vi "Get Spec.vi"(4 "NumRows":u32, 6 "Spec in":string[][](array[string]), 7 "Spec Ref.":refnum<vi>, 8 "error in":errorcluster caption="에러 입력(에러 없음)", 9 "Condition in":string[][](array[string]), 10 "Resolution in":string[][](array[string]), 11 "Func_ext":string) -> (0 "error out":errorcluster caption="에러 출력", 1 "Data Out":string[][](array[string]), 2 "Spec Out":string[][](array[string]), 3 "Func_ext Out":string, 5 "Spec (Default)":string[][](array[string]))   [LabVIEW 2020]
uses:
  Controls/Cmd_Var Data IO.ctl
  Variables/Global_Cal Info.vi
  Public/Polymorph/Data Class_2D Str.vi
panel:
  out "match spec":string[][](array[string])
  # "FUNC, FUNC_EXT, FUNC_CON, C1_VAL, C1_UNIT, RANGE_VAL, RANGE_UNIT"
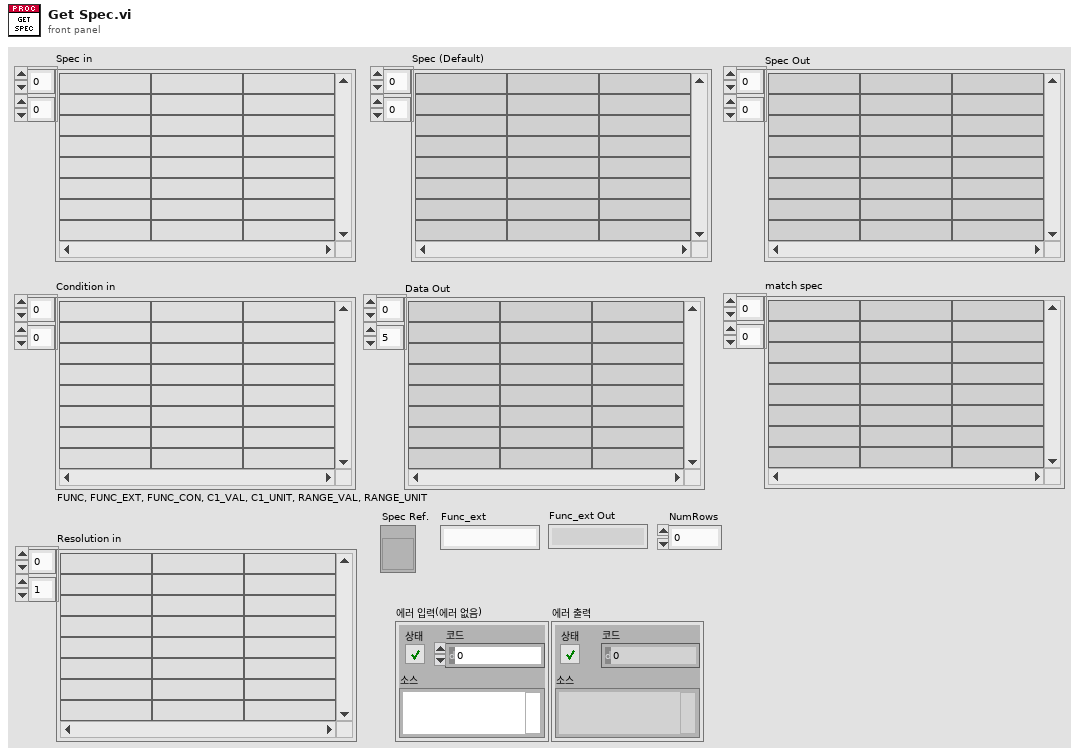
[diagram p1: front panel]
types:
  T1 = typedef "Cmd_Var Data IO.ctl" = enum16{"Condition", "Condition Default", "Condition_Temp", "Resolution", "Resolution Default", "Resolution Old", "Spec", "Spec Default", "Spec Old", "Spec Temp", "Result", "Result2", "Result3", "Result_Temp", "Result_ADJ", "Result_ADJ2", "STD1", "STD2", "STD3", "STD4", "STD5", "STD Temp", "CMC", "CMC Default"}
  T2 = cluster{"세부분류코드":string, "형식":string, "옵션":string, "측정기명":string, "EXCEL파일명":string, "TEMP":string}
  T3 = typedef "Clst_Cal Info Global.ctl" = cluster{"등록번호":string, "의뢰기관":string, "기기명":string, "제작회사":string, "형식":string, "기기번호":string, "소분류코드":string, "세부분류코드":string, "교정주기":string, "접수번호":string, "교정일자":string, "교정절차서 1":string, "교정절차서 2":string, "교정절차서 3":string, "접수확인자":string, "인증교정자":string, "기술책임자":string, "KOLAS 유무":string, "진행상태":string, "의뢰기관코드":string, "입고형태":string, "영문성적서?":bool, "합불판정?":bool, "부록?":bool, "절차서번호 1":string, "절차서번호 2":string, "절차서번호 3":string, "교정방식":string, "부서명":string}
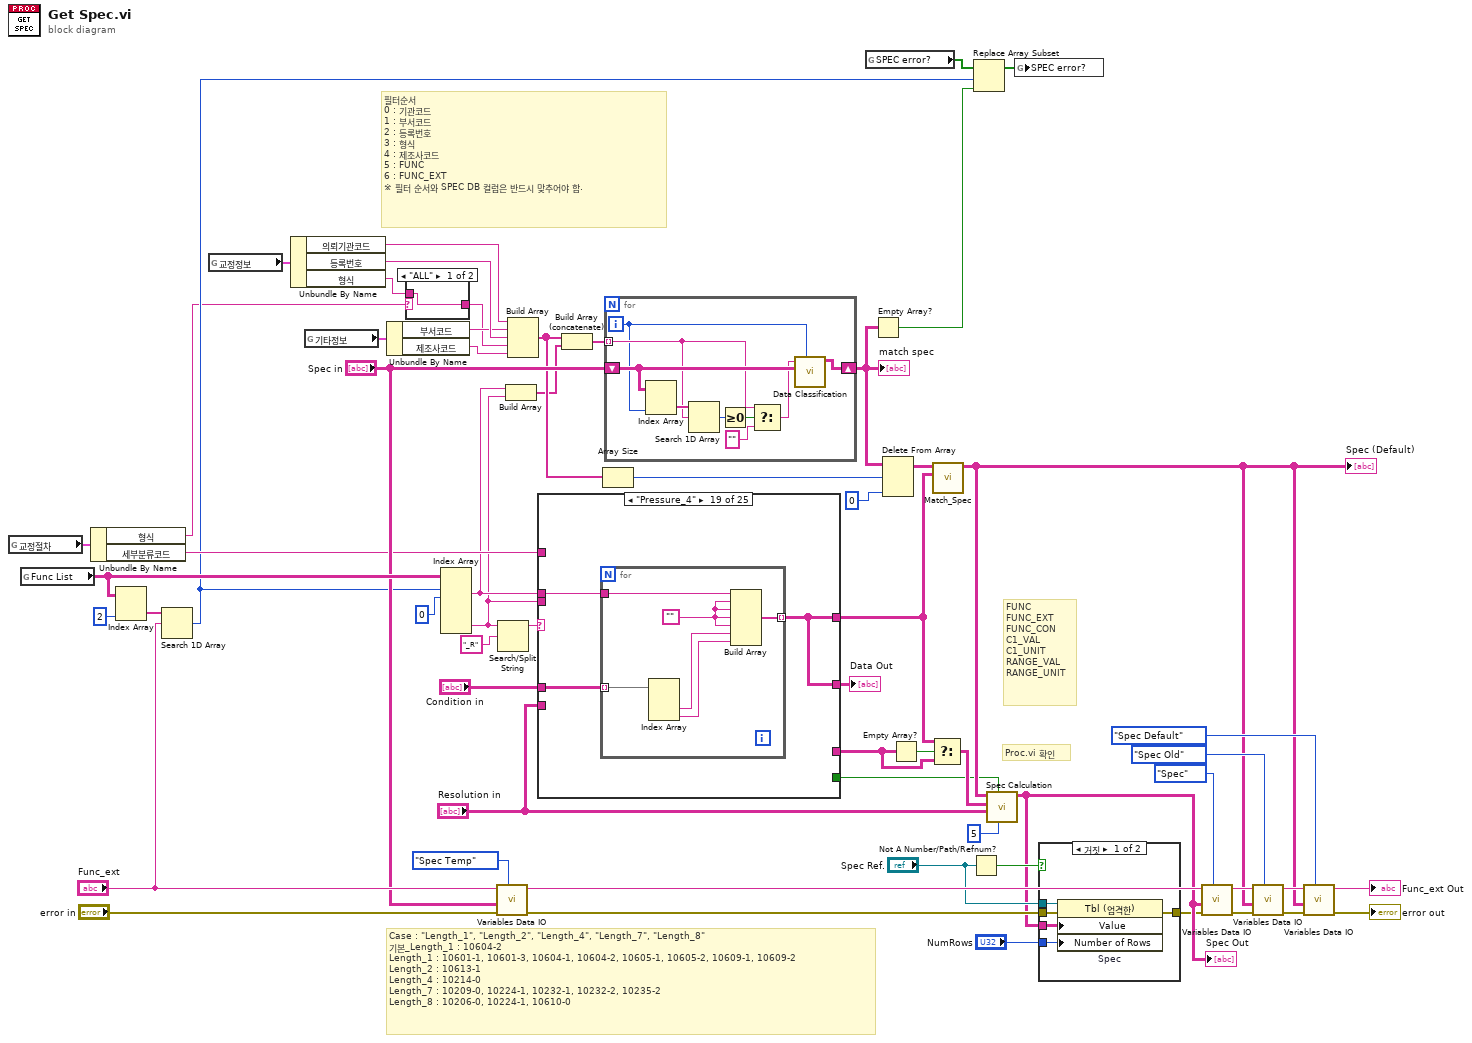
[diagram p0: block diagram]
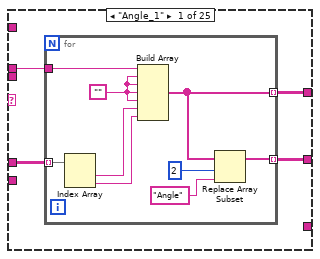
[diagram p4: hidden frame]
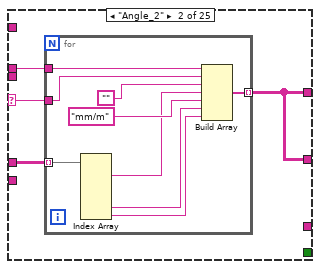
[diagram p5: hidden frame]
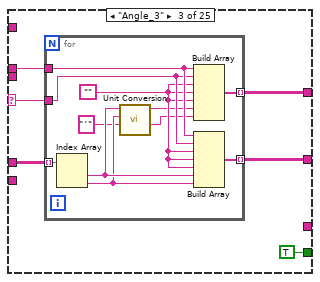
[diagram p6: hidden frame]
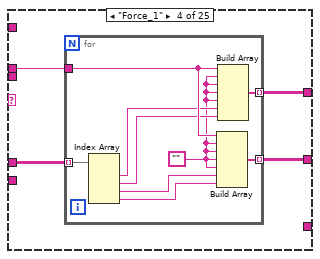
[diagram p7: hidden frame]
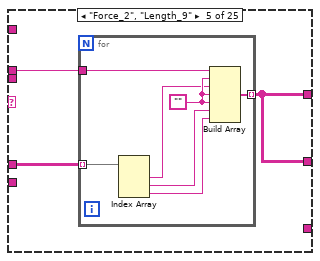
[diagram p8: hidden frame]
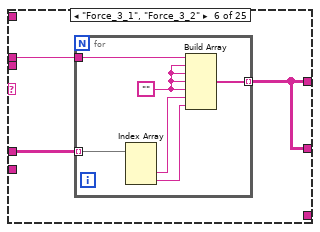
[diagram p9: hidden frame]
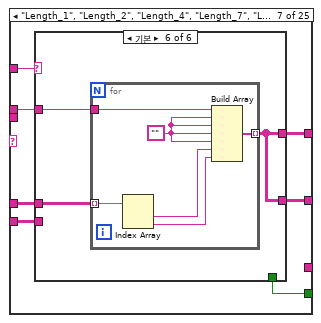
[diagram p10: hidden frame]
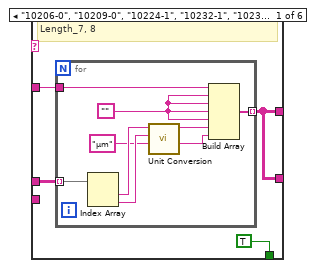
[diagram p11: hidden frame]
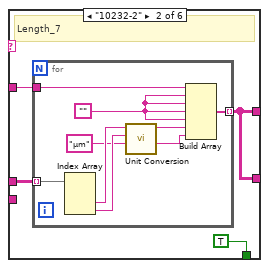
[diagram p12: hidden frame]
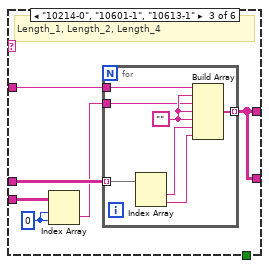
[diagram p13: hidden frame]
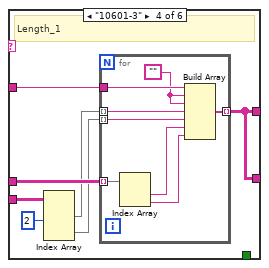
[diagram p14: hidden frame]
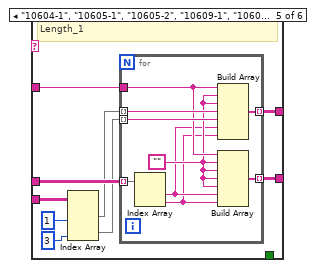
[diagram p15: hidden frame]
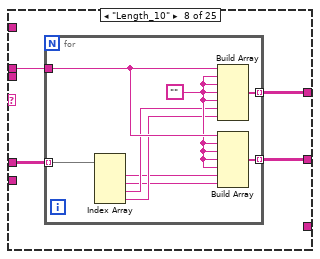
[diagram p16: hidden frame]
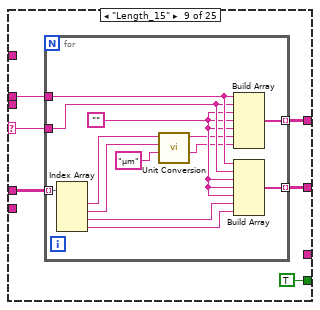
[diagram p17: hidden frame]
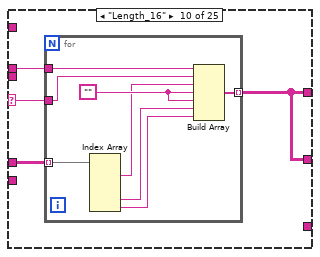
[diagram p18: hidden frame]
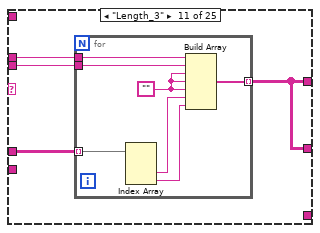
[diagram p19: hidden frame]
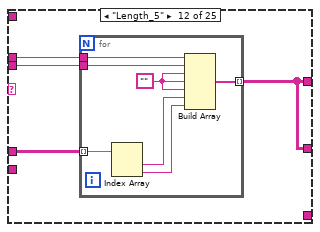
[diagram p20: hidden frame]
diagram:
  # "Proc.vi 확인"
  # "Case : \"Length_1\", \"Length_2\", \"Length_4\", \"Length_7\", \"Length_8\" \n기본_Length_1 : 10604-2\nLength_1 : 10601-1, 10601-3, 10604-1, 10604-2, 10605-1, 10605-2, 10609-1, 10609-2\nLength_2 : 10613-1\nLength_4 : 10214-0\nLength_7 : 10209-0, 10224-1, 10232-1, 10232-2, 10235-2\nLength_8 : 10206-0, 10224-1, 10610-0"
  # "필터순서\n0 : 기관코드\n1 : 부서코드\n2 : 등록번호\n3 : 형식\n4 : 제조사코드\n5 : FUNC\n6 : FUNC_EXT\n※ 필터 순서와 SPEC DB 컬럼은 반드시 맞추어야 함."
  # "FUNC\nFUNC_EXT\nFUNC_CON\nC1_VAL\nC1_UNIT\nRANGE_VAL\nRANGE_UNIT"
  n1 = global read "Global_Cal Info.vi" "교정절차"() -> (w59:T2)
  n2 = global read "Global_Cal Info.vi" "Func List"() -> (w48:string[][])
  n3 = Unbundle By Name(w59) -> ("형식"=w2:string, "세부분류코드"=w30:string)
  n4 = Index Array(array=w48, index (col)=2 ("비활성화된 인덱스 (열)")) -> (element=w50:string[])  [unwired: 1 in]
  n5 = Search 1D Array(1D array=w50, element="Func_ext") -> (index of element=w6:i32)  [unwired: 1 in]
  n6 = global read "Global_Cal Info.vi" "교정정보"() -> (w60:T3)
  n7 = Unbundle By Name(w60) -> ("의뢰기관코드"=w20:string, "등록번호"=w26:string, "형식"=w1:string)
  n8 = global read "Global_Cal Info.vi" "기타정보"() -> (w25:cluster{"부서코드":string, "제조사코드":string})
  n9 = Unbundle By Name(w25) -> ("부서코드"=w24:string, "제조사코드"=w23:string)
  n10 = case shown="\"ALL\"" w2 {
    selector: w2 -> [_ w62]
    tunnel: [w61 w62] -> w3
    tunnel: w1 -> [w61 _]
    frame "ALL" {
    }
    frame Default {
    }
  }
  n11 = Index Array(array=w48, index (row) #1=w6, index (col) #1=0 ("비활성화된 인덱스 (열)")) -> (element #1=w19:string, element #3=w18:string)  [unwired: 4 in, 1 out]
  n12 = call "Variables Data IO.vi"("Select"=Cmd_Var_Data_IO."Spec Temp", "error in"="error in", "Data In"="Spec in", "Func_ext"="Func_ext") -> ("error out"=w38:errorcluster, "Func_ext Out"=w36:string)  [unwired: 5 in, 1 out]
  n13 = Search/Split String(string=w18, search string/char (-)="_R" ("검색 문자열/문자 (-)")) -> (substring before match=w32:string)  [unwired: 1 in, 2 out]
  n14 = Build Array(w19, w18) -> (w16:string[])
  n15 = Build Array(w20, w24, w26, w3, w23) -> (w21:string[])
  n16 = case shown="\"Pressure_4\"" w32 {
    selector: w32 -> [_ w77 w92 _ _ _ _ _ w242 w259 _ _ w294 _ w322 _ _ _ _ w415 w431 w446 w462 w478 _]
    tunnel: "Condition in" -> [w66 w79 w94 w109 w121 w131 w144 w229 w244 w261 w273 w284 w296 w310 w324 w332 w342 w354 w405 w417 w433 w448 w464 w480 w494]
    tunnel: w19 -> [w65 w78 w93 w108 w120 w130 w143 w228 w243 w260 w272 w283 w295 w309 w323 w331 w341 w353 w404 w416 w432 w447 w463 w479 w493]
    tunnel: [w64 w76 w89 w107 w119 w129 w142 w227 w240 w258 w271 w282 w293 w307 w321 w330 w340 w351 w403 w413 w430 w443 w461 w476 w492] -> w13
    tunnel: [w63 w76 w91 w106 w119 w129 w139 w226 w241 w258 w271 w282 w293 w308 w321 w330 w340 w350 w403 w414 w430 w445 w461 w475 w492] -> w31
    tunnel: w30 -> [_ _ _ _ _ _ w140 _ _ _ _ _ _ _ _ _ _ w352 _ _ _ _ _ _ _]
    tunnel: "Resolution in" -> [_ _ _ _ _ _ w141 _ _ _ _ _ _ _ _ _ _ _ _ _ _ _ _ w477 _]
    tunnel: w18 -> [_ _ _ _ _ _ _ _ _ _ w270 w281 _ _ _ _ _ _ _ _ _ _ _ _ _]
    tunnel: [_ _ TRUE _ _ _ w138 _ TRUE _ _ _ TRUE _ _ _ _ _ _ _ TRUE TRUE _ _ _] -> w4
    tunnel: [_ _ _ _ _ _ _ _ _ _ _ _ _ _ _ _ _ _ _ w412 _ _ w460 _ _] -> w11
    frame "Angle_1" {
      n17 = for {
        tunnel: w66 -> [w75] mode=indexing
        tunnel: [w70] -> w64 mode=indexing
        tunnel: w65 -> [w74]
        tunnel: [w69] -> w63 mode=indexing
        w71 = ""
        n18 = Index Array(array=w75) -> (element #1=w72:string, element #2=w73:string)  [unwired: 2 in]
        n19 = Build Array(w74, w71, w71, w71, w71, w72, w73) -> (w70:string[])
        n20 = Replace Array Subset(array=w70, new element="Angle" ("새 원소/부분배열"), index=2 ("인덱스")) -> (w69:string[])
      }
    }
    frame "Angle_2" {
      n21 = for {
        tunnel: w79 -> [w88] mode=indexing
        tunnel: [w87] -> w76 mode=indexing
        tunnel: w78 -> [w86]
        tunnel: w77 -> [w85]
        n22 = Index Array(array=w88) -> (element #1=w82:string, element #5=w80:string, element #6=w81:string)  [unwired: 6 in, 3 out]
        n23 = Build Array(w86, w85, "", w82, "mm/m" ("원소"), w80, w81) -> (w87:string[])
      }
    }
    frame "Angle_3" {
      n24 = for {
        tunnel: w94 -> [w105] mode=indexing
        tunnel: [w104] -> w89 mode=indexing
        tunnel: w93 -> [w103]
        tunnel: [w102] -> w91 mode=indexing
        tunnel: w92 -> [w101]
        w100 = ""
        n25 = Index Array(array=w105) -> (element #1=w97:string, element #2=w96:string)  [unwired: 2 in]
        n26 = call "Unit Conversion.vi"("환산단위"="´", "입력단위"=w96, "입력값"=w97) -> ("환산단위"=w98:string, "환산값 (string)"=w99:string)  [unwired: 3 in, 4 out]
        n27 = Build Array(w103, w101, w100, w100, w100, w99, w98) -> (w104:string[])
        n28 = Build Array(w103, w101, w100, w100, w100, w97, w96) -> (w102:string[])
      }
    }
    frame "Force_1" {
      n29 = for {
        tunnel: w109 -> [w118] mode=indexing
        tunnel: [w117] -> w107 mode=indexing
        tunnel: w108 -> [w115]
        tunnel: [w116] -> w106 mode=indexing
        w110 = ""
        n30 = Index Array(array=w118) -> (element #1=w112:string, element #2=w111:string, element #3=w114:string, element #4=w113:string)  [unwired: 4 in]
        n31 = Build Array(w115, w110, w110, w110, w110, w114, w113) -> (w116:string[])
        n32 = Build Array(w115, w110, w110, w110, w110, w112, w111) -> (w117:string[])
      }
    }
    frame "Force_2", "Length_9" {
      n33 = for {
        tunnel: w121 -> [w128] mode=indexing
        tunnel: [w127] -> w119 mode=indexing
        tunnel: w120 -> [w126]
        w125 = ""
        n34 = Index Array(array=w128) -> (element #1=w124:string, element #2=w123:string, element #3=w122:string)  [unwired: 3 in]
        n35 = Build Array(w126, w125, w124, w125, w125, w123, w122) -> (w127:string[])
      }
    }
    frame "Force_3_1", "Force_3_2" {
      n36 = for {
        tunnel: w131 -> [w137] mode=indexing
        tunnel: [w136] -> w129 mode=indexing
        tunnel: w130 -> [w135]
        w132 = ""
        n37 = Index Array(array=w137) -> (element #2=w133:string, element #3=w134:string)  [unwired: 3 in, 1 out]
        n38 = Build Array(w135, w132, w132, w132, w132, w133, w134) -> (w136:string[])
      }
    }
    frame "Length_1", "Length_2", "Length_4", "Length_7", "Length_8" {
      n39 = case shown="기본" w140 {
        tunnel: w144 -> [w148 w161 w176 w190 w207 w219]
        tunnel: w143 -> [w147 w160 w175 w189 w206 w218]
        tunnel: [w146 w159 w171 w184 w205 w217] -> w142
        tunnel: w141 -> [_ _ w174 w188 w204 _]
        tunnel: [w146 w159 w171 w184 w199 w217] -> w139
        tunnel: [TRUE TRUE _ _ _ _] -> w138
        frame "10206-0", "10209-0", "10224-1", "10232-1", "10235-2", "10610-0" {
          # "Length_7, 8"
          n40 = for {
            tunnel: w148 -> [w157] mode=indexing
            tunnel: [w156] -> w146 mode=indexing
            tunnel: w147 -> [w155]
            w154 = ""
            n41 = Index Array(array=w157) -> (element #1=w153:string, element #2=w152:string)  [unwired: 2 in]
            n42 = call "Unit Conversion.vi"("환산단위"="μm", "입력단위"=w152, "입력값"=w153) -> ("환산단위"=w149:string, "환산값 (string)"=w150:string)  [unwired: 3 in, 4 out]
            n43 = Build Array(w155, w154, w154, w154, w154, w150, w149) -> (w156:string[])
          }
        }
        frame "10232-2" {
          # "Length_7"
          n44 = for {
            tunnel: w161 -> [w170] mode=indexing
            tunnel: [w169] -> w159 mode=indexing
            tunnel: w160 -> [w168]
            w167 = ""
            n45 = Index Array(array=w170) -> (element #2=w166:string, element #3=w165:string)  [unwired: 3 in, 1 out]
            n46 = call "Unit Conversion.vi"("환산단위"="μm", "입력단위"=w165, "입력값"=w166) -> ("환산단위"=w162:string, "환산값 (string)"=w163:string)  [unwired: 3 in, 4 out]
            n47 = Build Array(w168, w167, w167, w167, w167, w163, w162) -> (w169:string[])
          }
        }
        frame "10214-0", "10601-1", "10613-1" {
          w173 = 0 ("인덱스 (행)")
          # "Length_1, Length_2, Length_4"
          n48 = Index Array(array=w174, index (row)=w173, index (col)=w173) -> (element=w172:string)
          n49 = for {
            tunnel: w176 -> [w183] mode=indexing
            tunnel: [w182] -> w171 mode=indexing
            tunnel: w175 -> [w181]
            tunnel: w172 -> [w177]
            w178 = ""
            n50 = Index Array(array=w183) -> (element #1=w179:string, element #2=w180:string)  [unwired: 2 in]
            n51 = Build Array(w181, w178, w177, w178, w178, w179, w180) -> (w182:string[])
          }
        }
        frame "10601-3" {
          # "Length_1"
          n52 = Index Array(array=w188, index (col) #1=2 ("비활성화된 인덱스 (열)")) -> (element #1=w186:string[], element #2=w185:string[])  [unwired: 3 in]
          n53 = for {
            tunnel: w190 -> [w198] mode=indexing
            tunnel: [w197] -> w184 mode=indexing
            tunnel: w189 -> [w196]
            tunnel: w186 -> [w192] mode=indexing
            tunnel: w185 -> [w191] mode=indexing
            w193 = ""
            n54 = Index Array(array=w198) -> (element #1=w194:string, element #2=w195:string)  [unwired: 2 in]
            n55 = Build Array(w196, w193, w193, w192, w191, w194, w195) -> (w197:string[])
          }
        }
        frame "10604-1", "10605-1", "10605-2", "10609-1", "10609-2" {
          # "Length_1"
          n56 = Index Array(array=w204, index (col) #1=1 ("비활성화된 인덱스 (열)"), index (col) #2=3 ("인덱스 (열)")) -> (element #1=w202:string[], element #2=w201:string[])  [unwired: 2 in]
          n57 = for {
            tunnel: w207 -> [w216] mode=indexing
            tunnel: [w215] -> w205 mode=indexing
            tunnel: w206 -> [w212]
            tunnel: w202 -> [w214] mode=indexing
            tunnel: w201 -> [w213] mode=indexing
            tunnel: [w208] -> w199 mode=indexing
            w211 = ""
            n58 = Index Array(array=w216) -> (element #1=w210:string, element #2=w209:string)  [unwired: 2 in]
            n59 = Build Array(w212, w211, w211, w214, w213, w210, w209) -> (w215:string[])
            n60 = Build Array(w212, w211, w211, w211, w211, w210, w209) -> (w208:string[])
          }
        }
        frame Default {
          n61 = for {
            tunnel: w219 -> [w225] mode=indexing
            tunnel: [w224] -> w217 mode=indexing
            tunnel: w218 -> [w223]
            w221 = ""
            n62 = Index Array(array=w225) -> (element #1=w220:string, element #2=w222:string)  [unwired: 2 in]
            n63 = Build Array(w223, w221, w221, w221, w221, w220, w222) -> (w224:string[])
          }
        }
      }
    }
    frame "Length_10" {
      n64 = for {
        tunnel: w229 -> [w238] mode=indexing
        tunnel: [w237] -> w227 mode=indexing
        tunnel: w228 -> [w236]
        tunnel: [w235] -> w226 mode=indexing
        w234 = ""
        n65 = Index Array(array=w238) -> (element #1=w231:string, element #2=w230:string, element #3=w233:string, element #4=w232:string)  [unwired: 4 in]
        n66 = Build Array(w236, w234, w234, w234, w234, w233, w232) -> (w237:string[])
        n67 = Build Array(w236, w234, w234, w234, w234, w231, w230) -> (w235:string[])
      }
    }
    frame "Length_15" {
      n68 = for {
        tunnel: w244 -> [w257] mode=indexing
        tunnel: [w256] -> w240 mode=indexing
        tunnel: w243 -> [w255]
        tunnel: [w254] -> w241 mode=indexing
        tunnel: w242 -> [w253]
        w252 = ""
        n69 = Index Array(array=w257) -> (element #1=w249:string, element #2=w248:string, element #3=w251:string, element #4=w250:string)  [unwired: 4 in]
        n70 = call "Unit Conversion.vi"("환산단위"="μm", "입력단위"=w248, "입력값"=w249) -> ("환산단위"=w245:string, "환산값 (string)"=w246:string)  [unwired: 3 in, 4 out]
        n71 = Build Array(w255, w253, w252, w252, w252, w246, w245) -> (w256:string[])
        n72 = Build Array(w255, w253, w252, w252, w252, w251, w250) -> (w254:string[])
      }
    }
    frame "Length_16" {
      n73 = for {
        tunnel: w261 -> [w269] mode=indexing
        tunnel: [w268] -> w258 mode=indexing
        tunnel: w260 -> [w267]
        tunnel: w259 -> [w266]
        w265 = ""
        n74 = Index Array(array=w269) -> (element #1=w262:string, element #4=w264:string, element #5=w263:string)  [unwired: 5 in, 2 out]
        n75 = Build Array(w267, w266, w262, w265, w265, w264, w263) -> (w268:string[])
      }
    }
    frame "Length_3" {
      n76 = for {
        tunnel: w273 -> [w280] mode=indexing
        tunnel: [w279] -> w271 mode=indexing
        tunnel: w272 -> [w278]
        tunnel: w270 -> [w274]
        w275 = ""
        n77 = Index Array(array=w280) -> (element #2=w276:string, element #3=w277:string)  [unwired: 3 in, 1 out]
        n78 = Build Array(w278, w274, w275, w275, w275, w276, w277) -> (w279:string[])
      }
    }
    frame "Length_5" {
      n79 = for {
        tunnel: w284 -> [w291] mode=indexing
        tunnel: [w290] -> w282 mode=indexing
        tunnel: w283 -> [w289]
        tunnel: w281 -> [w285]
        w286 = ""
        n80 = Index Array(array=w291) -> (element #1=w287:string, element #2=w288:string)  [unwired: 2 in]
        n81 = Build Array(w289, w285, w286, w286, w286, w287, w288) -> (w290:string[])
      }
    }
    frame "Length_6_1", "Length_6_2" {
      n82 = for {
        tunnel: w296 -> [w303] mode=indexing
        tunnel: w295 -> [w306]
        tunnel: w294 -> [w305]
        tunnel: [w302] -> w293 mode=indexing
        w304 = ""
        n83 = Index Array(array=w303) -> (element #1=w301:string, element #2=w300:string)  [unwired: 2 in]
        n84 = call "Unit Conversion.vi"("환산단위"="μm" ("원소"), "입력단위"=w300, "입력값"=w301) -> ("환산단위"=w297:string, "환산값 (string)"=w299:string)  [unwired: 3 in, 4 out]
        n85 = Build Array(w306, w305, w304, w304, w304, w299, w297) -> (w302:string[])
      }
    }
    frame "Magnification_1" {
      n86 = for {
        tunnel: w310 -> [w320] mode=indexing
        tunnel: [w319] -> w308 mode=indexing
        tunnel: w309 -> [w314]
        tunnel: [w315] -> w307 mode=indexing
        w313 = ""
        n87 = Index Array(array=w320, index #1=2 ("인덱스")) -> (element #1=w317:string, element #2=w318:string, element #3=w312:string, element #4=w311:string)  [unwired: 3 in]
        n88 = Build Array(w314, w313, w313, w313, w313, w312, w311) -> (w315:string[])
        n89 = Build Array(w314, w313, w313, w313, w313, w317, w318) -> (w319:string[])
      }
    }
    frame "Mass_1_1", "Mass_1_2", "Mass_1_3" {
      n90 = for {
        tunnel: w324 -> [w329] mode=indexing
        tunnel: [w328] -> w321 mode=indexing
        tunnel: w323 -> [w327]
        tunnel: w322 -> [w326]
        w325 = ""
        n91 = Build Array (concatenate)(w327, w326, w325, w325, w325, w329) -> (w328:string[])
      }
    }
    frame "Mass_2_1" {
      n92 = for {
        tunnel: w332 -> [w339] mode=indexing
        tunnel: [w338] -> w330 mode=indexing
        tunnel: w331 -> [w337]
        w334 = ""
        n93 = Index Array(array=w339, index #1=4 ("인덱스")) -> (element #1=w335:string, element #2=w336:string)  [unwired: 1 in]
        n94 = Build Array(w337, w334, w334, w334, w334, w335, w336) -> (w338:string[])
      }
    }
    frame "Mass_2_2" {
      n95 = for {
        tunnel: w342 -> [w349] mode=indexing
        tunnel: [w348] -> w340 mode=indexing
        tunnel: w341 -> [w347]
        w345 = ""
        n96 = Index Array(array=w349, index #1=3 ("인덱스")) -> (element #1=w344:string, element #3=w346:string)  [unwired: 2 in, 1 out]
        n97 = Build Array(w347, w345, w345, w345, w345, w344, w346) -> (w348:string[])
      }
    }
    frame "Pressure_1", "Pressure_2", "Pressure_3" {
      n98 = case shown="기본" w352 {
        tunnel: w354 -> [w355 w376 w391]
        tunnel: w353 -> [w356 w375 w390]
        tunnel: [w358 w374 w389] -> w351
        tunnel: [w357 w373 w388] -> w350
        frame "20409-0" {
          n99 = for {
            tunnel: [w368] -> w358 mode=indexing
            tunnel: w356 -> [w361]
            tunnel: [w360] -> w357 mode=indexing
            tunnel: w355 -> [w367] mode=indexing
            w359 = ""
            n100 = Index Array(array=w367, index #1=4 ("인덱스"), index #3=1 ("인덱스"), index #4=3 ("인덱스")) -> (element #1=w370:string, element #2=w371:string, element #3=w364:string, element #4=w362:string)  [unwired: 1 in]
            n101 = Search and Replace String(input string=w364, search string="-" ("검색 문자열")) -> (result string=w363:string)  [unwired: 6 in, 3 out]
            n102 = Build Array(w361, w359, w359, w359, w359, w370, w371) -> (w368:string[])
            n103 = Build Array(w361, w359, w359, w359, w359, w363, w362) -> (w360:string[])
          }
        }
        frame "20412-1", "20412-2", "20412-3" {
          n104 = for {
            tunnel: w376 -> [w387] mode=indexing
            tunnel: [w383] -> w374 mode=indexing
            tunnel: w375 -> [w382]
            tunnel: [w378] -> w373 mode=indexing
            w377 = ""
            n105 = Index Array(array=w387, index #1=6 ("인덱스"), index #3=3 ("인덱스")) -> (element #1=w384:string, element #2=w385:string, element #3=w380:string, element #5=w379:string)  [unwired: 3 in, 1 out]
            n106 = Build Array(w382, w377, w377, w377, w377, w384, w385) -> (w383:string[])
            n107 = Build Array(w382, w377, w377, w377, w377, w380, w379) -> (w378:string[])
          }
        }
        frame Default {
          n108 = for {
            tunnel: w391 -> [w402] mode=indexing
            tunnel: [w398] -> w389 mode=indexing
            tunnel: w390 -> [w397]
            tunnel: [w393] -> w388 mode=indexing
            w392 = ""
            n109 = Index Array(array=w402, index #1=4 ("인덱스"), index #3=1 ("인덱스")) -> (element #1=w399:string, element #2=w400:string, element #3=w395:string, element #5=w394:string)  [unwired: 3 in, 1 out]
            n110 = Build Array(w397, w392, w392, w392, w392, w399, w400) -> (w398:string[])
            n111 = Build Array(w397, w392, w392, w392, w392, w395, w394) -> (w393:string[])
          }
        }
      }
    }
    frame "Pressure_4" {
      n112 = for {
        tunnel: w405 -> [w411] mode=indexing
        tunnel: [w410] -> w403 mode=indexing
        tunnel: w404 -> [w409]
        w408 = ""
        n113 = Index Array(array=w411) -> (element #2=w406:string, element #3=w407:string)  [unwired: 3 in, 1 out]
        n114 = Build Array(w409, w408, w408, w408, w408, w406, w407) -> (w410:string[])
      }
    }
    frame "Squareness_1" {
      n115 = for {
        tunnel: w417 -> [w428] mode=indexing
        tunnel: [w427] -> w413 mode=indexing
        tunnel: w416 -> [w423]
        tunnel: [w426] -> w414 mode=indexing
        tunnel: w415 -> [w422]
        tunnel: [w418] -> w412 mode=indexing
        w421 = ""
        n116 = Index Array(array=w428) -> (element #2=w425:string, element #3=w424:string, element #4=w420:string, element #5=w419:string)  [unwired: 5 in, 1 out]
        n117 = Build Array(w423, w422, w421, w421, w421, w425, w424) -> (w427:string[])
        n118 = Build Array(w423, w422, w421, w421, w421, w425, w424) -> (w426:string[])
        n119 = Build Array(w423, w422, w421, w421, w421, w420, w419) -> (w418:string[])
      }
    }
    frame "Flatness_1", "Squareness_2" {
      n120 = for {
        tunnel: w433 -> [w442] mode=indexing
        tunnel: [w441] -> w430 mode=indexing
        tunnel: w432 -> [w440]
        tunnel: w431 -> [w439]
        n121 = Index Array(array=w442) -> (element #1=w438:string, element #3=w435:string, element #4=w436:string)  [unwired: 4 in, 1 out]
        n122 = Build Array(w440, w439, "", w435, w436, w438, "μm" ("원소")) -> (w441:string[])
      }
    }
    frame "Straightness_1" {
      n123 = for {
        tunnel: w448 -> [w459] mode=indexing
        tunnel: [w458] -> w443 mode=indexing
        tunnel: w447 -> [w457]
        tunnel: [w456] -> w445 mode=indexing
        tunnel: w446 -> [w455]
        w454 = ""
        n124 = Index Array(array=w459) -> (element #1=w451:string, element #2=w450:string)  [unwired: 2 in]
        n125 = call "Unit Conversion.vi"("환산단위"="mm", "입력단위"=w450, "입력값"=w451) -> ("환산단위"=w452:string, "환산값 (string)"=w453:string)  [unwired: 3 in, 4 out]
        n126 = Build Array(w457, w455, w454, w454, w454, w453, w452) -> (w458:string[])
        n127 = Build Array(w457, w455, w454, w454, w454, w451, w450) -> (w456:string[])
      }
    }
    frame "Torque_1" {
      n128 = for {
        tunnel: w464 -> [w473] mode=indexing
        tunnel: [w474] -> w461 mode=indexing
        tunnel: w463 -> [w472]
        tunnel: w462 -> [w471]
        tunnel: [w467] -> w460 mode=indexing
        w470 = ""
        n129 = Index Array(array=w473) -> (element #1=w465:string, element #2=w466:string, element #3=w469:string, element #4=w468:string)  [unwired: 4 in]
        n130 = Build Array(w472, w471, w470, w470, w470, w465, w466) -> (w474:string[])
        n131 = Build Array(w472, w471, w470, w470, w470, w469, w468) -> (w467:string[])
      }
    }
    frame "Torque_2" {
      n132 = for {
        tunnel: w480 -> [w490] mode=indexing
        tunnel: [w491] -> w476 mode=indexing
        tunnel: w479 -> [w487]
        tunnel: w478 -> [w486]
        tunnel: w477 -> [w489] mode=indexing
        tunnel: [w481] -> w475 mode=indexing
        w485 = ""
        n133 = Index Array(array=w490) -> (element #3=w484:string, element #4=w483:string)  [unwired: 4 in, 2 out]
        n134 = Index Array(array=w489) -> (element=w488:string)  [unwired: 1 in]
        n135 = Build Array(w487, w486, w488, w485, w485, w484, w483) -> (w491:string[])
        n136 = Build Array(w487, w486, "시계" ("원소"), w485, w485, w484, w483) -> (w481:string[])
      }
    }
    frame Default {
      n137 = for {
        tunnel: w494 -> [w500] mode=indexing
        tunnel: [w499] -> w492 mode=indexing
        tunnel: w493 -> [w498]
        w495 = ""
        n138 = Index Array(array=w500) -> (element #1=w496:string, element #2=w497:string)  [unwired: 2 in]
        n139 = Build Array(w498, w495, w495, w495, w495, w496, w497) -> (w499:string[])
      }
    }
  }
  "Data Out" <- w31
  n140 = Build Array (concatenate)(w21, w16) -> (w17:string[])
  n141 = Array Size(array=w21) -> (size(s)=w22:i32)
  n142 = for {
    tunnel: w17 -> [w505] mode=indexing
    shift-right: [w506] -> w9
    shift-left: "Spec in" -> [w509]
    i -> [w503]
    n143 = Index Array(array=w509, index (col)=w503) -> (element=w508:string[])  [unwired: 1 in]
    n144 = Search 1D Array(1D array=w508, element=w505) -> (index of element=w507:i32)  [unwired: 1 in]
    n145 = Greater Or Equal To 0?(x=w507) -> (x >= 0?=w502:bool)
    n146 = Select(t=w505, s=w502, f="") -> (s? t:f=w504:string)
    n147 = call-poly "Data Classification.vi"("인덱스"=w503, "DATA 입력"=w509, "검색 문자열"=w504) -> ("DATA 출력"=w506:string[][])  [unwired: 4 in, 4 out]
  }
  "match spec" <- w9
  n148 = global read "Global_Cal Info.vi" "SPEC error?"() -> (w8:bool[])
  n149 = Empty Array?(array=w9) -> (empty?=w5:bool)
  n150 = Delete From Array(array=w9, length=w22, index (col)=0 ("비활성화된 인덱스 (열)")) -> (array with subset deleted=w57:string[][])  [unwired: 1 in, 1 out]
  n151 = Empty Array?(array=w11) -> (empty?=w14:bool)
  n152 = Select(t=w13, s=w14, f=w11) -> (s? t:f=w12:string[][])
  n153 = call "Match_Spec.vi"("DATA IN"=w13, "SPEC IN"=w57) -> ("Spec Out"=w40:string[][])  [unwired: 7 in, 2 out]
  "Spec (Default)" <- w40
  n154 = Not A Number/Path/Refnum?(number/path/refnum="Spec Ref.") -> (NaN/Path/Refnum?=w28:bool)
  n155 = Replace Array Subset(array=w8, new element=w5, index=w6) -> (w7:bool[])
  n156 = call "Spec Calculation.vi"("기준값 열번호"=5 ("열번호(기준값)"), "0기준?"=w4, "Resolution"="Resolution in", "Condition in"=w12, "Spec Default"=w40) -> ("Spec out"=w15:string[][])  [unwired: 5 in, 1 out]
  "Spec Out" <- w15
  n157 = global write "Global_Cal Info.vi" "SPEC error?"(w7) -> ()
  n158 = case shown="거짓" w28 {
    tunnel: [w514 w515] -> w10
    tunnel: "NumRows" -> [w513 _]
    tunnel: w15 -> [w512 _]
    tunnel: w38 -> [w511 w515]
    tunnel: "Spec Ref." -> [w510 _]
    frame False {
      n159 = property on="Spec" class="Tbl (엄격한)"(reference=w510, error in=w511, "Value"=w512, "Number of Rows"=w513) -> (error out=w514:errorcluster)  [unwired: 1 out]
    }
    frame True {
    }
  }
  n160 = call "Variables Data IO.vi"("Select"=Cmd_Var_Data_IO."Spec", "error in"=w10, "Data In"=w15, "Func_ext"=w36) -> ("error out"=w46:errorcluster, "Func_ext Out"=w44:string)  [unwired: 5 in, 1 out]
  n161 = call "Variables Data IO.vi"("Select"=Cmd_Var_Data_IO."Spec Old", "error in"=w46, "Data In"=w40, "Func_ext"=w44) -> ("error out"=w45:errorcluster, "Func_ext Out"=w43:string)  [unwired: 5 in, 1 out]
  n162 = call "Variables Data IO.vi"("Select"=Cmd_Var_Data_IO."Spec Default", "error in"=w45, "Data In"=w40, "Func_ext"=w43) -> ("error out"=→"error out":errorcluster, "Func_ext Out"=→"Func_ext Out":string)  [unwired: 5 in, 1 out]
